vi "Group data by data type.vi"(9 "Update UI count indicators":bool, 11 "Raw data":T1) -> (1 "POI data":T1, 2 "Miniscan data":T1, 3 "Number of selected ROI per type":cluster{"# sel POI":i32, "# sel MSCN":i32})   [LabVIEW 2020]
uses:
  xcontrol/Interface VIs/Interface typedefs/Interface-Data array.ctl
  xcontrol/Interface VIs/Interface typedefs/Interface-Data format definition.ctl
  xcontrol/Typedefs/Xctl-XY data type definition.ctl
  xcontrol/Typedefs/Xctrl-ROI type enum.ctl
  Global variables/gl_Functional Imaging-Global variables.vi
  xcontrol/XGrapher.xctl
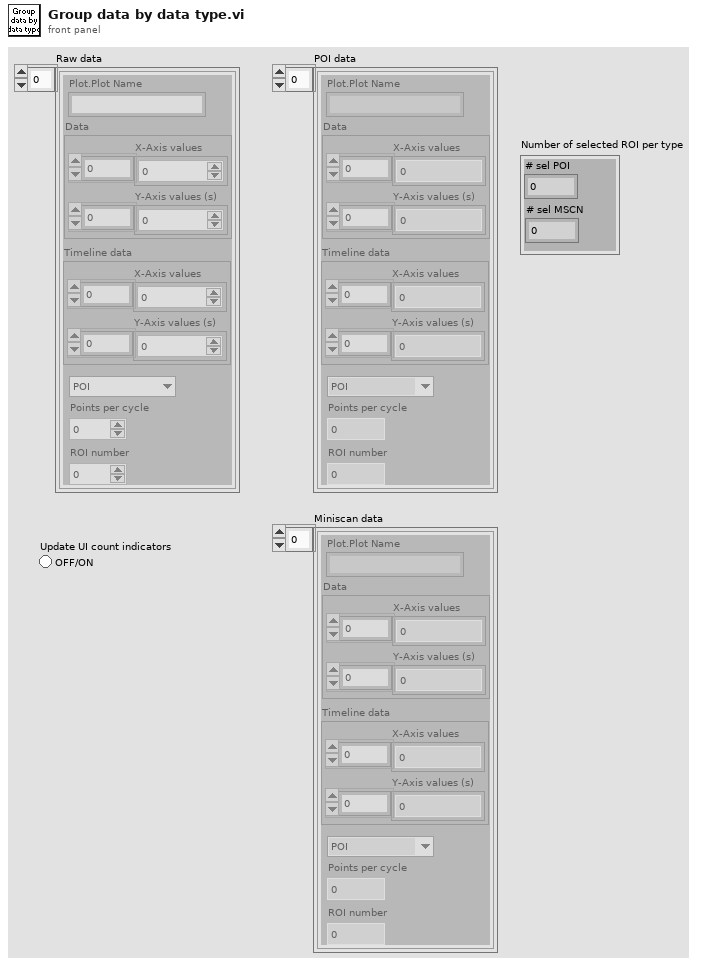
[diagram p1: front panel]
types:
  T1 = typedef "Interface-Data array.ctl" = T2[]
  T2 = typedef "Interface-Data format definition.ctl" = cluster{"Plot.Plot Name":string, "Data":T3, "Timeline data":T3, "Type":T4, "Points per cycle":u16, "ROI number":u16}
  T3 = typedef "XGrapher.xctl/Xctl-XY data type definition.ctl" = cluster{"X-Axis values":sgl[], "Y-Axis values (s)":sgl[]}
  T4 = typedef "Xctrl-ROI type enum.ctl" = enum16{"POI", "Mini-scan", "Group"}
  T5 = typedef "Functional Imging UI Refs.ctl" = cluster{"Menu ref":refnum<k9>, "Image control":refnum<vi>, "VI ref":refnum<vi>, "XGrapher":refnum<vi>, "Smoothing":refnum<vi>, "POI Averaging":refnum<vi>, "Normalize":refnum<vi>, "POI data points in each trial":refnum<vi>, "Channel":refnum<vi>, "Experiment data folder path":refnum<vi>, "[ROI vis]":refnum<vi>, "[Groups] visbl":T6, "Group Name":refnum<vi>, "POI index":refnum<vi>, "Trial No.":refnum<vi>, "Intensity Zoom":refnum<vi>, "Trial Cursor Enabled":refnum<vi>, "Number of Trials (ind 1)":refnum<vi>, "Number of Trials (ind 2)":refnum<vi>, "MiniScans Available":refnum<vi>, "POI Available":refnum<vi>, "Defer graph updates":refnum<vi>, "Waveform selector":refnum<vi>, "#of selected POI":refnum<vi>, "#of selected MiniScans":refnum<vi>, "#of selected groups":refnum<vi>, "Max Z-Projection":refnum<vi>, "Z-Plane Selector":refnum<vi>, "Index of miniscan point to visualise":refnum<vi>, "ROI vis. mode":refnum<vi>, "Total # of points":refnum<vi>, "Index of group clicked on":refnum<vi>, "Pane 1":refnum<vi>, "Pane 2":refnum<vi>, "Pane 3":refnum<vi>, "Pane 4":refnum<vi>, "Pane 5":refnum<vi>, "Pane 6":refnum<vi>, "Deselect all ROI":refnum<vi>, "Deselect all groups":refnum<vi>}
  T6 = typedef "Groups array referecne.ctl" = refnum<vi>
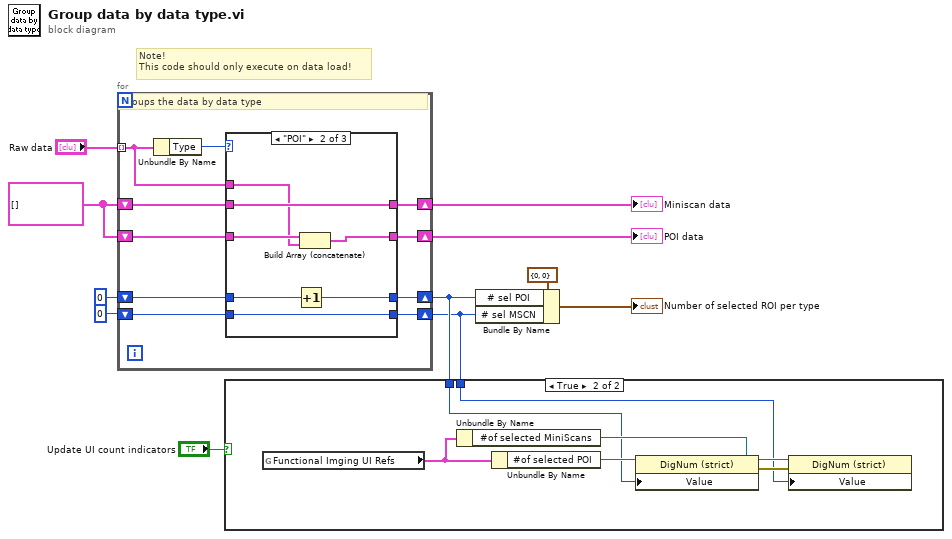
[diagram p0: block diagram]
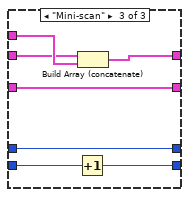
[diagram p4: hidden frame]
diagram:
  w5 = T1 [] ("Raw data out")
  # "Note!\nThis code should only execute on data load!"
  n1 = for {
    tunnel: "Raw data" -> [w19] mode=indexing
    shift-right: [w20] -> w10
    shift-left: w5 -> [w18]
    shift-right: [w17] -> w11
    shift-left: w5 -> [w16]
    shift-right: [w15] -> w7
    shift-left: 0 -> [w14]
    shift-right: [w12] -> w8
    shift-left: 0 -> [w13]
    # "Groups the data by data type"
    n2 = Unbundle By Name(w19) -> ("Type"=w21:T4)
    n3 = case shown="\"POI\"" w21 {
      tunnel: w19 -> [_ w29 w39]
      tunnel: [w24 w32 w38] -> w20
      tunnel: w18 -> [w24 w31 w38]
      tunnel: [w25 w30 w37] -> w17
      tunnel: w16 -> [w25 w30 w36]
      tunnel: [w22 w28 w35] -> w15
      tunnel: w14 -> [w22 w28 w34]
      tunnel: [w23 w26 w33] -> w12
      tunnel: w13 -> [w23 w27 w33]
      frame Default {
      }
      frame "POI" {
        n4 = Increment(x=w27) -> (x+1=w26:i32)
        n5 = Build Array (concatenate)(w31, w29) -> (w32:T1)
      }
      frame "Mini-scan" {
        n6 = Increment(x=w34) -> (x+1=w35:i32)
        n7 = Build Array (concatenate)(w36, w39) -> (w37:T1)
      }
    }
  }
  "Miniscan data" <- w11
  "POI data" <- w10
  n8 = case shown="True" "Update UI count indicators" {
    tunnel: w8 -> [_ w41]
    tunnel: w7 -> [_ w40]
    frame False {
    }
    frame True {
      n9 = global read "gl_Functional Imaging-Global variables.vi" "Functional Imging UI Refs"() -> (w42:T5)
      n10 = Unbundle By Name(w42) -> ("#of selected MiniScans"=w44:refnum<vi>)
      n11 = Unbundle By Name(w42) -> ("#of selected POI"=w45:refnum<vi>)
      n12 = property on="Property Node" class="DigNum (strict)"(reference=w45, "Value"=w41) -> (error out=w43:errorcluster)  [unwired: 1 in, 1 out]
      n13 = property on="Property Node" class="DigNum (strict)"(reference=w44, error in=w43, "Value"=w40) -> ()  [unwired: 2 out]
    }
  }
  n14 = Bundle By Name(cluster=cluster{"# sel POI":i32, "# sel MSCN":i32} {"# sel POI"=0, "# sel MSCN"=0} ("Cluster"), "# sel POI"=w8, "# sel MSCN"=w7) -> (→"Number of selected ROI per type":cluster{"# sel POI":i32, "# sel MSCN":i32})
